vi "Transfer GUID.vi"() -> (3 "GUID":string="88fcfa75-3196-4ae9-a459-f2e46a72afc7")   [LabVIEW 2017, in "Data Sharing Framework System Explorer.lvlib"]
uses:
  Data Sharing Framework System Explorer.lvlib
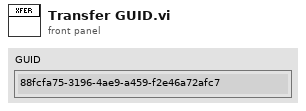
[diagram p1: front panel]
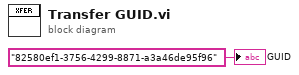
[diagram p0: block diagram]
diagram:
  "GUID" <- "82580ef1-3756-4299-8871-a3a46de95f96" ("Data Sharing Framework")
